vi "BoxBegin.vi"(8 "error in (no error)":errorcluster) -> (0 "error out":errorcluster)   [LabVIEW 2023]
uses:
  <vilib>/Rock Robotics/SystemInterfaces/DIO/FPGA_DIOChannel.ctl
  <vilib>/Rock Robotics/WPI/ThirdParty/REV Robotics/REVLib/Typedef/Spark MAX Sensor Type.ctl
  <vilib>/Rock Robotics/WPI/ThirdParty/REV Robotics/REVLib/Typedef/Spark MAX Idle Mode.ctl
  <vilib>/Rock Robotics/WPI/ThirdParty/REV Robotics/REVLib/Typedef/Spark MAX Motor Type.ctl
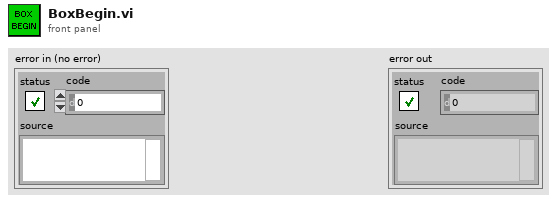
[diagram p1: front panel]
types:
  T1 = typedef "FPGA_DIOChannel.ctl" = enum8{"DIO 0", "DIO 1", "DIO 2", "DIO 3", "DIO 4", "DIO 5", "DIO 6", "DIO 7", "DIO 8", "DIO 9", "DIO MXP 0", "DIO MXP 1", "DIO MXP 2", "DIO MXP 3", "DIO MXP 4", "DIO MXP 5", "DIO MXP 6", "DIO MXP 7", "DIO MXP 8", "DIO MXP 9", "DIO MXP 10", "DIO MXP 11", "DIO MXP 12", "DIO MXP 13", "DIO MXP 14", "DIO MXP 15", "SPI Port CS1", "SPI Port CS2", "SPI Port CS3", "SPI Port MISO", "SPI Port MOSI", "Invalid"}
  T2 = typedef "Spark MAX Sensor Type.ctl" = enum16{"No Sensor", "Hall Sensor", "Encoder", "-Not Available-", "Analog", "Alternate Encoder", "Duty Cycle"}
  T3 = typedef "Spark MAX Idle Mode.ctl" = enum16{"Coast", "Brake"}
  T4 = typedef "Spark MAX Motor Type.ctl" = enum16{"Brushed", "Brushless"}
  T5 = typedef "WPI_DigitalInputDevRef.ctl" = cluster{"DevStatus":errorcluster, "DIO Channel":T1}
  T6 = typedef "WPI_MotorControlDeviceRef.ctl" = cluster{"DeviceStatus":errorcluster, "Type":T7, "PWM":cluster{"PWM Channel":T8, "DeadBand":T9}, "CAN":cluster{"Device Number":u8, "SetOutput VI Ref":variant, "GetOutput VI Ref":variant, "Enable VI Ref":variant, "Disable VI Ref":variant, "Data":variant}, "Invert":bool, "DIO PWM":cluster{"PWM \"Enable\" Channel":T8, "DIOChannel":T1, "PWM Rate":dbl}}
  T7 = typedef "WPI_MotorControlType.ctl" = enum16{"PWM", "CAN", "DIO PWM"}
  T8 = typedef "FPGA_DIOPWMChannel.ctl" = enum8{"PWM 0", "PWM 1", "PWM 2", "PWM 3", "PWM 4", "PWM 5", "PWM 6", "PWM 7", "PWM 8", "PWM 9", "PWM MXP 0", "PWM MXP 1", "PWM MXP 2", "PWM MXP 3", "PWM MXP 4", "PWM MXP 5", "PWM MXP 6", "PWM MXP 7", "PWM MXP 8", "PWM MXP 9", "Invalid"}
  T9 = typedef "WPI_PWMDeadband.ctl" = cluster{"Name":string, "maxPositivePwm":i32, "minPositivePwm":i32, "centerPwm":i32, "maxNegativePwm":i32, "minNegativePwm":i32, "angularRange":u16}
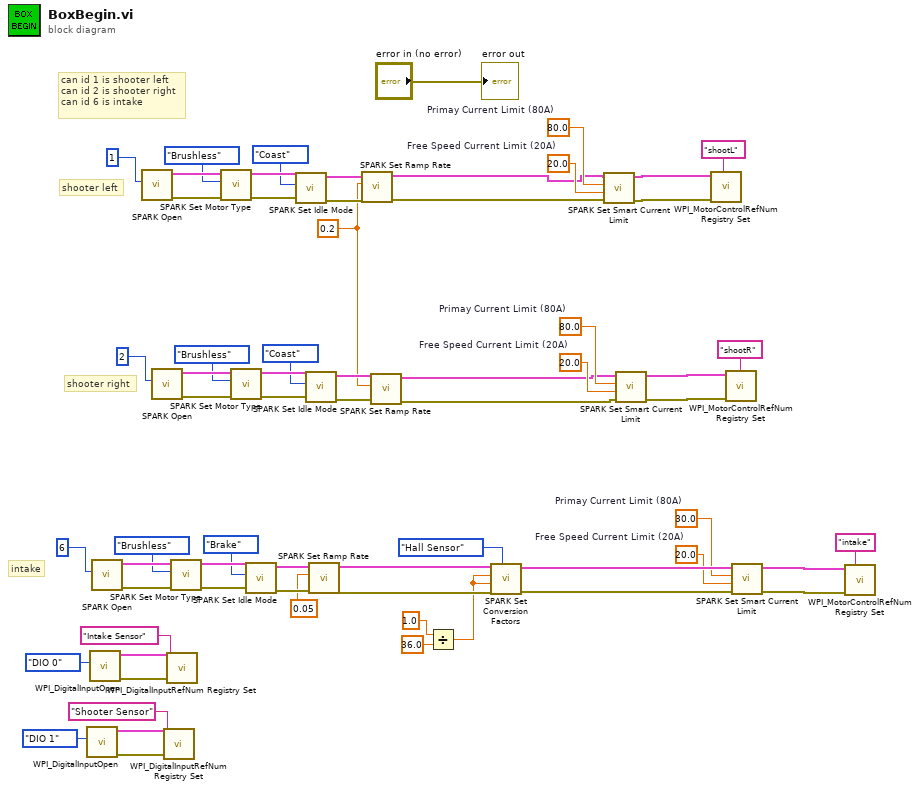
[diagram p0: block diagram]
diagram:
  w5 = 20.0  # Free Speed Current Limit (20A)
  w6 = 80.0  # Primay Current Limit (80A)
  w11 = 20.0  # Free Speed Current Limit (20A)
  w12 = 80.0  # Primay Current Limit (80A)
  w13 = 20.0  # Free Speed Current Limit (20A)
  w14 = 30.0  # Primay Current Limit (80A)
  w35 = 0.2
  # "intake"
  # "shooter right"
  # "shooter left"
  # "can id 1 is shooter left\ncan id 2 is shooter right\ncan id 6 is intake"
  n1 = call <vilib>:"WPI_DigitalInputOpen.vi"("DIO Channel"=FPGA_DIOChannel."DIO 1") -> ("error out"=w22:errorcluster, "DigitalInputDevRef"=w21:T5)  [unwired: 9 in]
  n2 = call <vilib>:"WPI_DigitalInputOpen.vi"("DIO Channel"=FPGA_DIOChannel."DIO 0") -> ("error out"=w26:errorcluster, "DigitalInputDevRef"=w25:T5)  [unwired: 9 in]
  n3 = call <vilib>:"SPARK Open.vi"("Device Number"=6) -> ("error out"=w45:errorcluster, "MotorControlDeviceRef"=w47:T6)  [unwired: 9 in]
  n4 = call <vilib>:"SPARK Open.vi"("Device Number"=1) -> ("error out"=w61:errorcluster, "MotorControlDeviceRef"=w63:T6)  [unwired: 9 in]
  n5 = call <vilib>:"SPARK Open.vi"("Device Number"=2) -> ("error out"=w53:errorcluster, "MotorControlDeviceRef"=w55:T6)  [unwired: 9 in]
  n6 = call <vilib>:"WPI_DigitalInputRefNum Registry Set.vi"("error in (no error)"=w22, "refnum name"="Shooter Sensor", "DigitalInputDevRef"=w21) -> ()  [unwired: 7 in, 2 out]
  n7 = call <vilib>:"WPI_DigitalInputRefNum Registry Set.vi"("error in (no error)"=w26, "refnum name"="Intake Sensor", "DigitalInputDevRef"=w25) -> ()  [unwired: 7 in, 2 out]
  n8 = call <vilib>:"SPARK Set Motor Type.vi"("error in (no error)"=w45, "Motor Type"=Spark_MAX_Motor_Type."Brushless", "MotorControlDevRef"=w47) -> ("error out"=w44:errorcluster, "MotorControlDeviceRef"=w46:T6)  [unwired: 7 in]
  n9 = call <vilib>:"SPARK Set Motor Type.vi"("error in (no error)"=w61, "Motor Type"=Spark_MAX_Motor_Type."Brushless", "MotorControlDevRef"=w63) -> ("error out"=w60:errorcluster, "MotorControlDeviceRef"=w62:T6)  [unwired: 7 in]
  n10 = call <vilib>:"SPARK Set Motor Type.vi"("error in (no error)"=w53, "Motor Type"=Spark_MAX_Motor_Type."Brushless", "MotorControlDevRef"=w55) -> ("error out"=w52:errorcluster, "MotorControlDeviceRef"=w54:T6)  [unwired: 7 in]
  n11 = call <vilib>:"SPARK Set Idle Mode.vi"("error in (no error)"=w44, "Idle Mode"=Spark_MAX_Idle_Mode."Brake", "MotorControlDeviceRef in"=w46) -> ("error out"=w36:errorcluster, "MotorControlDeviceRef out"=w37:T6)  [unwired: 7 in]
  n12 = call <vilib>:"SPARK Set Idle Mode.vi"("error in (no error)"=w60, "Idle Mode"=Spark_MAX_Idle_Mode."Coast", "MotorControlDeviceRef in"=w62) -> ("error out"=w39:errorcluster, "MotorControlDeviceRef out"=w38:T6)  [unwired: 7 in]
  n13 = call <vilib>:"SPARK Set Idle Mode.vi"("error in (no error)"=w52, "Idle Mode"=Spark_MAX_Idle_Mode."Coast", "MotorControlDeviceRef in"=w54) -> ("error out"=w40:errorcluster, "MotorControlDeviceRef out"=w41:T6)  [unwired: 7 in]
  n14 = call <vilib>:"SPARK Set Ramp Rate.vi"("error in (no error)"=w36, "Seconds from neutral to full (0)"=0.05, "MotorControlDeviceRef in"=w37) -> ("error out"=w33:errorcluster, "MotorControlDeviceRef"=w32:T6)  [unwired: 7 in]
  n15 = call <vilib>:"SPARK Set Ramp Rate.vi"("error in (no error)"=w39, "Seconds from neutral to full (0)"=w35, "MotorControlDeviceRef in"=w38) -> ("error out"=w3:errorcluster, "MotorControlDeviceRef"=w4:T6)  [unwired: 7 in]
  n16 = call <vilib>:"SPARK Set Ramp Rate.vi"("error in (no error)"=w40, "Seconds from neutral to full (0)"=w35, "MotorControlDeviceRef in"=w41) -> ("error out"=w9:errorcluster, "MotorControlDeviceRef"=w10:T6)  [unwired: 7 in]
  n17 = Divide(x=1.0, y=36.0) -> (x/y=w28:dbl)
  n18 = call <vilib>:"SPARK Set Conversion Factors.vi"("Sensor Type (Hall Sensor)"=Spark_MAX_Sensor_Type."Hall Sensor", "error in (no error)"=w33, "Velocity Factor (1)"=w28, "Position Factor (1)"=w28, "MotorControlDeviceRef in"=w32) -> ("error out"=w15:errorcluster, "MotorControlDeviceRef out"=w18:T6)  [unwired: 5 in]
  n19 = call <vilib>:"SPARK Set Smart Current Limit.vi"("error in (no error)"=w3, "Free Speed Current Limit (20A)"=w5, "Primay Current Limit (80A)"=w6, "MotorControlDeviceRef in"=w4) -> ("error out"=w1:errorcluster, "MotorControlDeviceRef out"=w2:T6)  [unwired: 6 in]
  n20 = call <vilib>:"SPARK Set Smart Current Limit.vi"("error in (no error)"=w9, "Free Speed Current Limit (20A)"=w11, "Primay Current Limit (80A)"=w12, "MotorControlDeviceRef in"=w10) -> ("error out"=w7:errorcluster, "MotorControlDeviceRef out"=w8:T6)  [unwired: 6 in]
  n21 = call <vilib>:"WPI_MotorControlRefNum Registry Set.vi"("error in (no error)"=w1, "refnum name"="shootL", "MotorControlDevRef"=w2) -> ()  [unwired: 7 in, 2 out]
  n22 = call <vilib>:"WPI_MotorControlRefNum Registry Set.vi"("error in (no error)"=w7, "refnum name"="shootR", "MotorControlDevRef"=w8) -> ()  [unwired: 7 in, 2 out]
  n23 = call <vilib>:"SPARK Set Smart Current Limit.vi"("error in (no error)"=w15, "Free Speed Current Limit (20A)"=w13, "Primay Current Limit (80A)"=w14, "MotorControlDeviceRef in"=w18) -> ("error out"=w16:errorcluster, "MotorControlDeviceRef out"=w17:T6)  [unwired: 6 in]
  n24 = call <vilib>:"WPI_MotorControlRefNum Registry Set.vi"("error in (no error)"=w16, "refnum name"="intake", "MotorControlDevRef"=w17) -> ()  [unwired: 7 in, 2 out]
  "error out" <- "error in (no error)"
